vi "Read CSMStates with lvcsm Support.vi"(7 "Current Module(\"\" to generate a ID)":string, 8 "error in (no error)":errorcluster, 9 "Force?(F)":bool, 11 "CSM Name":string) -> (0 "Error out":errorcluster, 3 "Value":string[](array[string]))   [LabVIEW 2020]
uses:
  b7efc127-9b6c-49b9-9e9d-39643bcb625b.vi
  166189b3-b0ee-4f88-bea7-bb947d9812ee.vi
  <vilib>/Utility/config.llb/Open Config Data.vi
  <vilib>/Utility/Data Type/Get Type Information.vi
  <vilib>/Utility/config.llb/Read Key.vi
  <vilib>/Utility/config.llb/Read Key (Boolean).vi
  <vilib>/Utility/config.llb/Read Key (String).vi
  <userlib>/_NEVSTOP/Communicable State Machine(CSM)/Utility/CSM Data Type String.vi
  <vilib>/Utility/config.llb/Get Key Names.vi
  <vilib>/Utility/config.llb/Read Key (Path).vi
  <vilib>/Utility/config.llb/Read Key (I32).vi
  <vilib>/Utility/config.llb/Read Key (Double).vi
  <userlib>/_NEVSTOP/Communicable State Machine(CSM)/Utility/_openG/Array of VData to VCluster_csm.vi
  <vilib>/Utility/config.llb/Close Config Data.vi
  <userlib>/_NEVSTOP/Communicable State Machine(CSM)/_csmHelper/API/Create From VI Reference.vi
  <userlib>/_NEVSTOP/Communicable State Machine(CSM)/_csmHelper/Properties/Read States.vi
  <userlib>/_NEVSTOP/Communicable State Machine(CSM)/_csmHelper/API/Destroy.vi
  <vilib>/Utility/config.llb/Write Key.vi
  <vilib>/Utility/config.llb/Write Key (Boolean).vi
  <vilib>/Utility/config.llb/Remove Key.vi
  <vilib>/Utility/config.llb/Write Key (String).vi
  <vilib>/Utility/config.llb/Write Key (Path).vi
  <vilib>/Utility/config.llb/Write Key (I32).vi
  <vilib>/Utility/config.llb/Write Key (Double).vi
  <userlib>/_NEVSTOP/Communicable State Machine(CSM)/_csmHelper/CSM-Helper.lvclass
  <userlib>/_NEVSTOP/Communicable State Machine(CSM)/Communicable State Machine.lvlib
  <userlib>/_NEVSTOP/Communicable State Machine(CSM)/_csmHelper/lvcsmFile/lvcsm File Support.lvlib
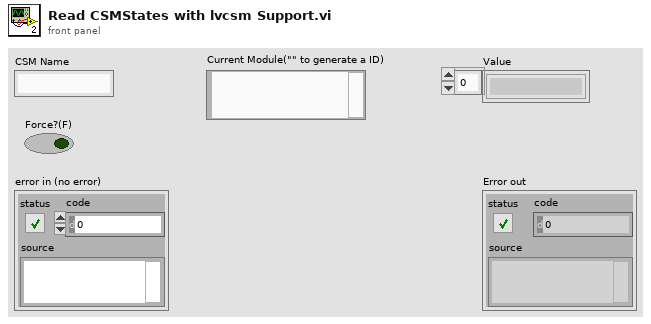
[diagram p1: front panel]
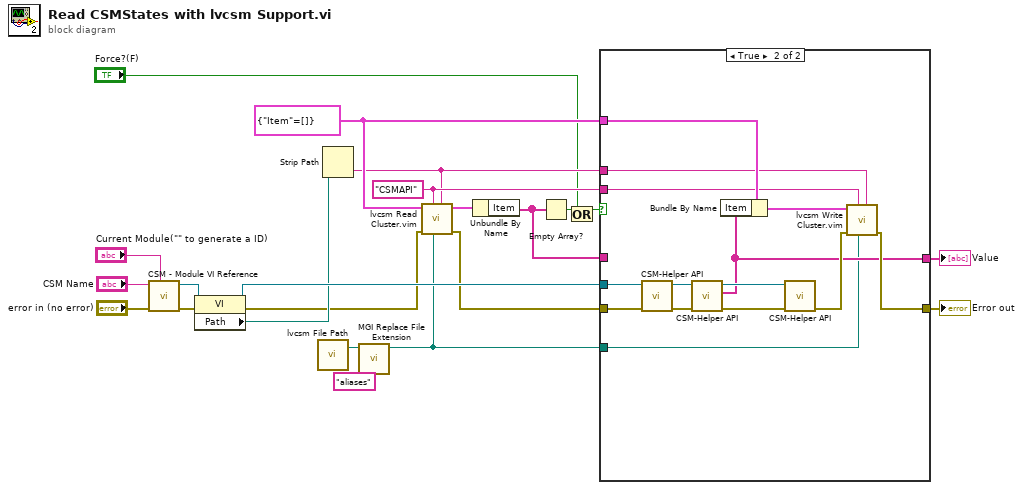
[diagram p0: block diagram]
diagram:
  w14 = cluster{"Item":string[]} {"Item"=[]}
  w13 = "CSMAPI" ("Section")
  n1 = call <userlib>:"CSM - Module VI Reference.vi"("Current Module(\"\" to generate a ID)"="Current Module(\"\" to generate a ID)", "error in (no error)"="error in (no error)", "CSM Name"="CSM Name") -> ("error out"=w22:errorcluster, "CSM Module VIRef"=w21:refnum<vi>)  [unwired: 7 in]
  n2 = property class="VI"(reference=w21, error in=w22) -> (reference out=w20:refnum<vi>, error out=w16:errorcluster, "Path"=w19:path)
  n3 = call <userlib>:"lvcsm File Path.vi"() -> ("appended path"=w3:path)  [unwired: 3 in]
  n4 = Strip Path(path=w19) -> (name=w12:string)  [unwired: 1 out]
  n5 = call <userlib>:"MGI Replace File Extension.vi"("New Extension (txt)"="aliases", "Path In"=w3) -> ("Path Out"=w1:path)  [unwired: 8 in, 1 out]
  n6 = call "lvcsm Read Cluster.vim"("sub-section(\"\")"=w12, "Config Path"=w1, "Section"=w13, "Error in"=w16, "Default Prototype"=w14) -> ("Error out"=w15:errorcluster, "Cluster (dup)"=w18:cluster{"Item":string[]})  [unwired: 5 in]
  n7 = Unbundle By Name(w18) -> ("Item"=w11:string[])
  n8 = Empty Array?(array=w11) -> (empty?=w17:bool)
  n9 = Or(x=w17, y="Force?(F)") -> (x .or. y?=w5:bool)
  n10 = case shown="True" w5 {
    tunnel: w15 -> [w24 w34]
    tunnel: w20 -> [_ w33]
    tunnel: [w24 w29] -> w10
    tunnel: w14 -> [_ w32]
    tunnel: w13 -> [_ w28]
    tunnel: w12 -> [_ w27]
    tunnel: [w23 w26] -> w6
    tunnel: w11 -> [w23 _]
    tunnel: w1 -> [_ w25]
    frame False {
    }
    frame True {
      n11 = call-poly <userlib>:"CSM-Helper API.vi"("error in (no error)"=w34, "VI"=w33) -> ("error out"=w36:errorcluster, "CSM-Helper.lvclass"=w35:refnum<class "CSM-Helper.lvclass">)  [unwired: 8 in]
      n12 = call-poly <userlib>:"CSM-Helper API.vi"("error in (no error)"=w36, "CSM-Helper in"=w35) -> ("error out"=w38:errorcluster, "Value"=w26:string[], "CSM-Helper out"=w37:refnum<class "CSM-Helper.lvclass">)  [unwired: 7 in]
      n13 = Bundle By Name(cluster=w32, "Item"=w26) -> (w31:cluster{"Item":string[]})
      n14 = call-poly <userlib>:"CSM-Helper API.vi"("error in (no error)"=w38, "CSM-Helper in"=w37) -> ("error out"=w30:errorcluster)  [unwired: 8 in, 1 out]
      n15 = call "lvcsm Write Cluster.vim"("sub-section(\"\")"=w27, "Config Path"=w25, "Section"=w28, "Error in"=w30, "Default Prototype"=w31) -> ("Error out"=w29:errorcluster)  [unwired: 6 in]
    }
  }
  "Error out" <- w10
  "Value" <- w6
